vi "Test shm log Event arrays LV.vi"(8 "error in (no error)":errorcluster, 11 "logevent_arrays_Ctl":T1) -> (0 "error out":errorcluster, 2 "function return":i32, 3 "logevent_arrays_Ctl out":T1)   [LabVIEW 2018, in "SALLV_Test.lvlib"]
doc: "int Test_shm_logEvent_arraysLV(Test_logevent_arraysLV *logevent_arrays_Ctl );"
uses:
  SALLV_Test.lvlib
  SALLV_Test.so
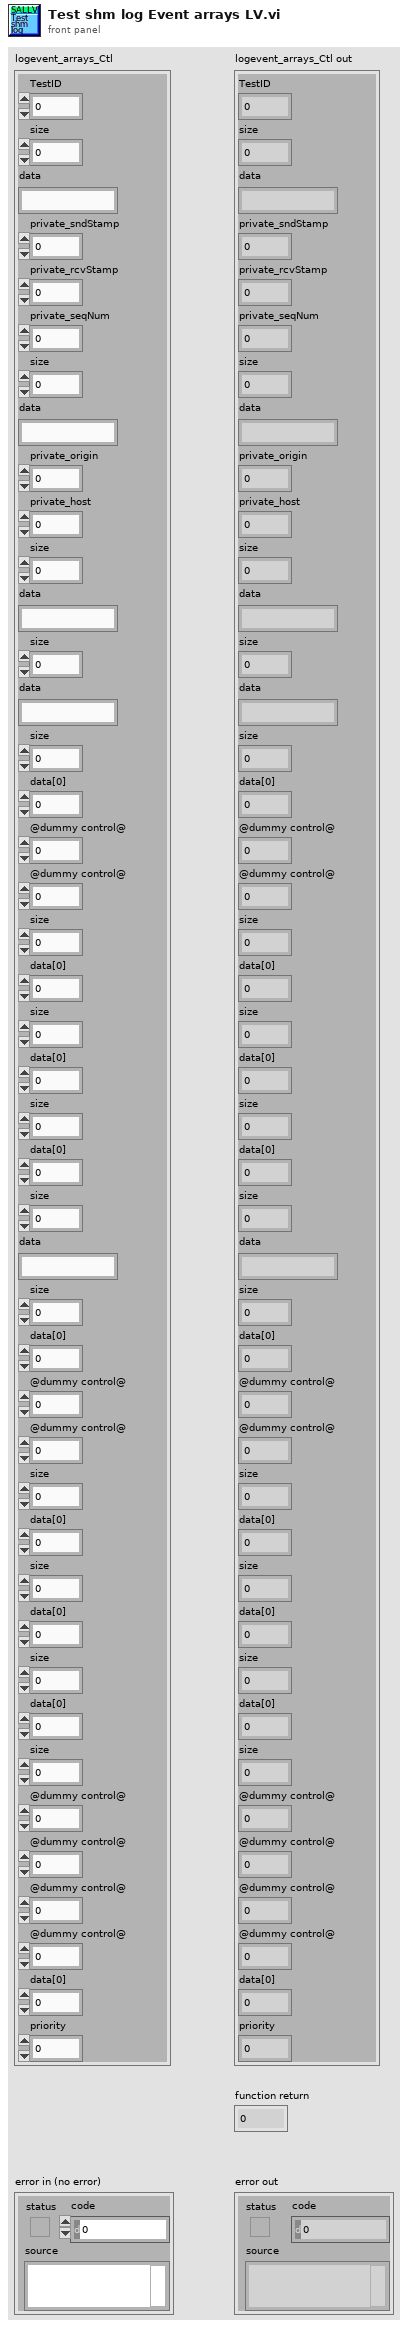
[diagram p1: front panel]
types:
  T1 = cluster{"TestID":i32, "size":i32, "data":string, "private_sndStamp":dbl, "private_rcvStamp":dbl, "private_seqNum":i32, "size":i32, "data":string, "private_origin":i32, "private_host":i32, "size":i32, "data":string, "size":i32, "data":string, "size":i32, "data[0]":i16, "@dummy control@":i8, "@dummy control@":i8, "size":i32, "data[0]":i32, "size":i32, "data[0]":i32, "size":i32, "data[0]":i32, "size":i32, "data":string, "size":i32, "data[0]":u16, "@dummy control@":i8, "@dummy control@":i8, "size":i32, "data[0]":u32, "size":i32, "data[0]":u32, "size":i32, "data[0]":sgl, "size":i32, "@dummy control@":i8, "@dummy control@":i8, "@dummy control@":i8, "@dummy control@":i8, "data[0]":dbl, "priority":i32}
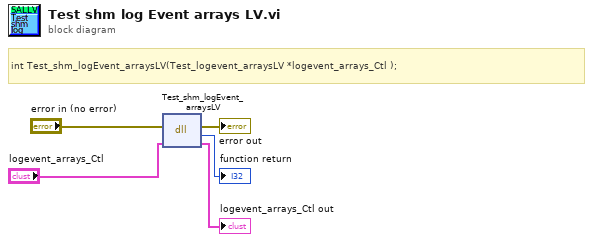
[diagram p0: block diagram]
diagram:
  # "int Test_shm_logEvent_arraysLV(Test_logevent_arraysLV *logevent_arrays_Ctl );"
  n1 = dll-call lib="home/ttsai/Documents/salTestLabViewApi/SALLV_Test/SALLV_Test.*" fn="Test_shm_logEvent_arraysLV"(error in="error in (no error)", "logevent_arrays_Ctl"="logevent_arrays_Ctl") -> (error out=→"error out":errorcluster, →"function return":i32, "logevent_arrays_Ctl"=→"logevent_arrays_Ctl out":T1)  [unwired: 2 in, 1 out]
